vi "UR Server 3.vi"() -> ()   [LabVIEW 2016]
panel:
  in  "stop":bool
  out "size(s)":i32
  out "data":string
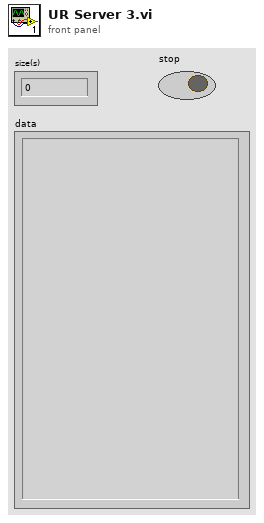
[diagram p1: front panel]
types:
  T1 = enum16{"Standard", "Buffered", "CRLF", "Immediate"}
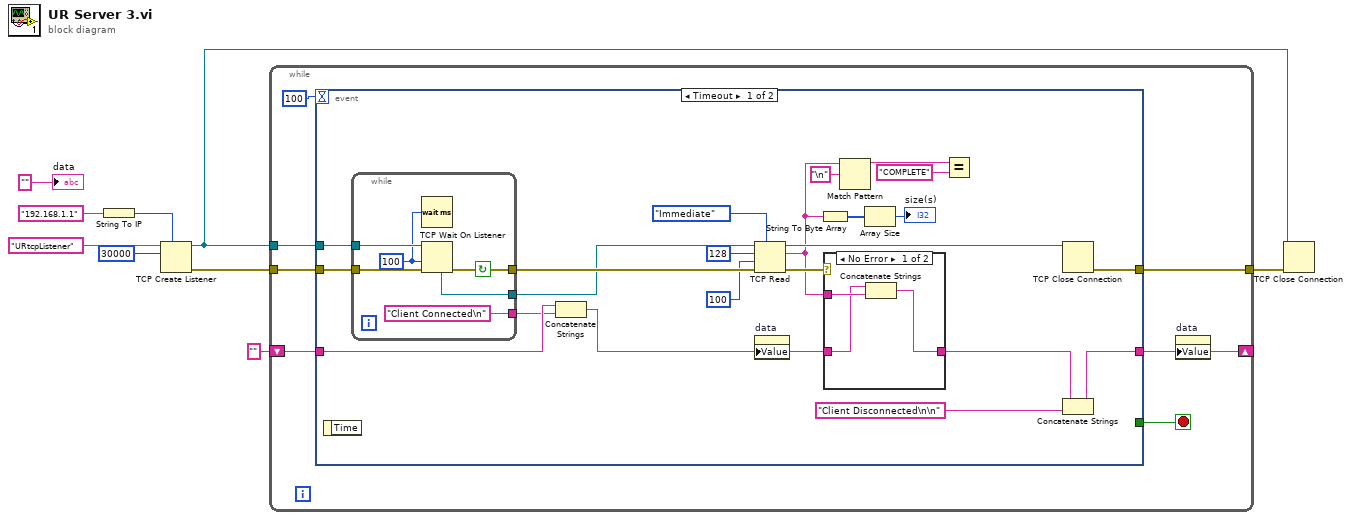
[diagram p0: block diagram]
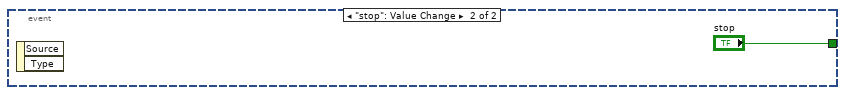
[diagram p3: hidden frame]
diagram:
  n1 = String To IP(1:"192.168.1.1" ("name")) -> (0:w7:u32)
  n2 = TCP Create Listener(7:w7, 10:u16 30000 ("remote port or service name"), 11:"URtcpListener" ("service name")) -> (0:w5:errorcluster, 3:w4:refnum<k5>)  [unwired: 2 in, 1 out]
  n3 = while {
    tunnel: w5 -> [w16]
    tunnel: w4 -> [w15]
    tunnel: [w14] -> w2
    shift-right: [w10] -> _
    shift-left: "" -> [w11]
    stop <- w12 stop-if-true
    n4 = event shown="[0] Timeout" {
      selector: _ -> [_ _]
      dyn-events: _ -> [_ _]
      timeout: 100 -> [_ _]
      tunnel: w16 -> [w38 _]
      tunnel: w15 -> [w37 _]
      tunnel: [w33 _] -> w14
      tunnel: [_ "stop"] -> w12
      tunnel: [w28 _] -> w10
      tunnel: w11 -> [w32 _]
      event Timeout {
        n5 = event-data() -> ()  [unwired: 1 in, 1 out]
        n6 = while {
          tunnel: w38 -> [w47]
          tunnel: [w45] -> w36
          tunnel: [w44] -> w35
          tunnel: w37 -> [w48]
          tunnel: ["Client Connected\n"] -> w30
          stop <- w45 continue-if-true
          w46 = 100 ("timeout ms (wait forever: -1)")
          n7 = Wait (ms)(milliseconds to wait=w46) -> ()  [unwired: 1 out]
          n8 = TCP Wait On Listener(8:w47, 9:w46, 11:w48) -> (0:w45:errorcluster, 4:w44:refnum<k5>)  [unwired: 1 in, 3 out]
        }
        n9 = Concatenate Strings(w32, w30) -> (w31:string)
        n10 = TCP Read(connection ID=w35, bytes to read=128, error in (no error)=w36, 7:T1."Immediate" ("mode (standard)"), 9:100 ("timeout ms (25000)")) -> (connection ID out=w34:refnum<k5>, data out=w20:string, error out=w26:errorcluster)
        n11 = property on="data" class="Str"("Value"=w31) -> ()  [unwired: 2 in, 2 out]
        n12 = String To Byte Array(string=w20) -> (unsigned byte array=w22:u8[])
        n13 = case shown="No Error" w26 {
          tunnel: w20 -> [w41 _]
          tunnel: [w40 w42] -> w29
          tunnel: w31 -> [w39 w42]
          frame No Error {
            n14 = Concatenate Strings(w39, w41) -> (w40:string)
          }
          frame Error {
          }
        }
        n15 = Match Pattern(string=w20, regular expression="\n") -> (before substring=w18:string)  [unwired: 1 in, 3 out]
        n16 = Array Size(array=w22) -> (size(s)=→"size(s)":i32)
        n17 = Equal?(x=w18, y="COMPLETE") -> ()  [unwired: 1 out]
        n18 = TCP Close Connection(connection ID=w34) -> (error out=w33:errorcluster)  [unwired: 2 in, 1 out]
        n19 = Concatenate Strings(w29, "Client Disconnected\n\n") -> (w28:string)
      }
      event "stop": Value Change {
        n20 = event-data() -> ()  [unwired: 1 in, 2 out]
      }
    }
    n21 = property on="data" class="Str"("Value"=w10) -> ()  [unwired: 2 in, 2 out]
  }
  n22 = TCP Close Connection(connection ID=w4, error in (no error)=w2) -> ()  [unwired: 1 in, 2 out]
  "data" <- "" ("data out")
